vi "CleanupTraces.vi"(8 "Baseline Rate":dbl=0.001, 9 "Spacing":dbl=100.0, 10 "decimating factor":i32=10, 11 "Traces in":waveform(i32)[](array[waveform])) -> (3 "Traces out":waveform(dbl)[](array[waveform]))   [LabVIEW 2012]
uses:
  <vilib>/Analysis/2dsp.llb/Decimate (continuous, DBL).vi
  <vilib>/Analysis/baseanly.llb/Mean (DBL).vi
  <vilib>/Analysis/NI_AALPro.lvlib
  <vilib>/Analysis/NI_AALBase.lvlib
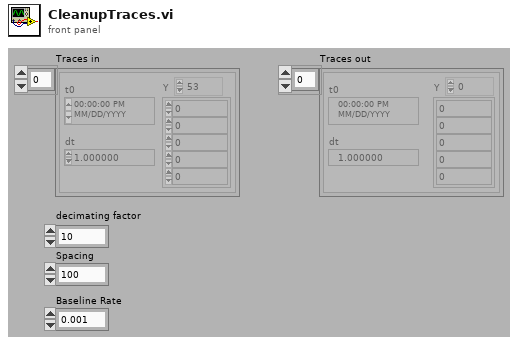
[diagram p1: front panel]
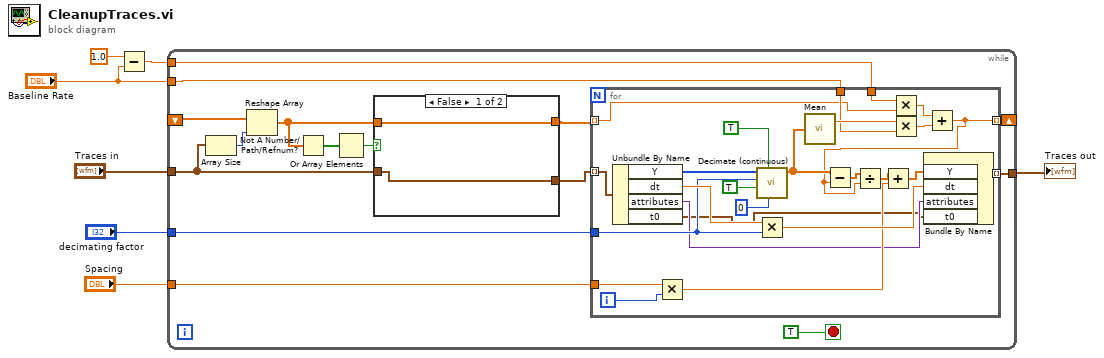
[diagram p0: block diagram]
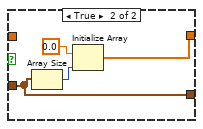
[diagram p2: hidden frame]
diagram:
  n1 = Subtract(x=1.0, y="Baseline Rate") -> (x-y=w1:dbl)
  n2 = while {
    tunnel: "Traces in" -> [w11]
    tunnel: "decimating factor" -> [w22]
    tunnel: "Spacing" -> [w21]
    tunnel: [w20] -> w4
    shift-right: [w18] -> _
    shift-left: _ -> [w17]
    tunnel: "Baseline Rate" -> [w15]
    tunnel: w1 -> [w14]
    stop <- TRUE stop-if-true
    n3 = Array Size(array=w11) -> (size(s)=w16:i32)
    n4 = Reshape Array(w17, w16) -> (w8:dbl[])
    n5 = Not A Number/Path/Refnum?(number/path/refnum=w8) -> (NaN/Path/Refnum?=w13:bool[])
    n6 = Or Array Elements(Boolean array=w13) -> (logical OR=w12:bool)
    n7 = case shown="False" w12 {
      tunnel: w11 -> [w23 w28]
      tunnel: [w23 w28] -> w10
      tunnel: [w24 w25] -> w9
      tunnel: w8 -> [w24 _]
      frame False {
      }
      frame True {
        n8 = Array Size(array=w28) -> (size(s)=w27:i32)
        n9 = Initialize Array(0.0, w27) -> (w25:dbl[])
      }
    }
    n10 = for {
      tunnel: w10 -> [w53] mode=indexing
      tunnel: w22 -> [w48]
      tunnel: w21 -> [w45]
      tunnel: [w42] -> w20 mode=indexing
      tunnel: [w29] -> w18 mode=indexing
      tunnel: w9 -> [w33] mode=indexing
      tunnel: w15 -> [w36]
      tunnel: w14 -> [w35]
      i -> [w46]
      n11 = Unbundle By Name(w53) -> ("Y"=w52:i32[], "dt"=w49:dbl, "attributes"=w31:variant, "t0"=w30:timestamp)
      n12 = Multiply(x=w45, y=w46) -> (x*y=w43:dbl)
      n13 = call-poly <vilib>:"Decimate (continuous).vi"("start index"=0, "reset"=TRUE, "averaging"=TRUE, "decimating factor"=w48, "X"=w52) -> ("Decimated Array"=w38:dbl[])  [unwired: 5 in, 1 out]
      n14 = Multiply(x=w49, y=w48) -> (x*y=w47:dbl)
      n15 = call-poly <vilib>:"Mean.vi"("X"=w38) -> ("mean"=w41:dbl)  [unwired: 1 out]
      n16 = Multiply(x=w35, y=w33) -> (x*y=w39:dbl)
      n17 = Multiply(x=w41, y=w36) -> (x*y=w40:dbl)
      n18 = Add(x=w39, y=w40) -> (x+y=w29:dbl)
      n19 = Subtract(x=w38, y=w29) -> (x-y=w34:dbl[])
      n20 = Divide(x=w34, y=w29) -> (x/y=w32:dbl[])
      n21 = Add(x=w32, y=w43) -> (x+y=w44:dbl[])
      n22 = Bundle By Name("Y"=w44, "dt"=w47, "attributes"=w31, "t0"=w30) -> (w42:waveform(dbl))  [unwired: 1 in]
    }
  }
  "Traces out" <- w4
